vi "Cache.Status.Fglb.vi"(5 "SystemIdx":i32, 7 "Action (get)":T4=enum."get", 8 "error in (no error)":errorcluster, 9 "CheckStatusData":T2, 10 "NewData":T1 {"Values" format="%.3f"}, 11 "Changeover":string) -> (0 "error out":errorcluster, 2 "Data":T3 {"NewData"."Values" format="%.3f"})   [LabVIEW 2016]
uses:
  Cache.Status.Fglb.Action.ctl
  Cache.Status.Fglb.Data.ctl
  Drivers/PLC/LowLevel/PLC.DataBlock.PCcheckstatus.ctl
  Drivers/PLC/LowLevel/PLC.DataBlock.PLCvalues.ctl
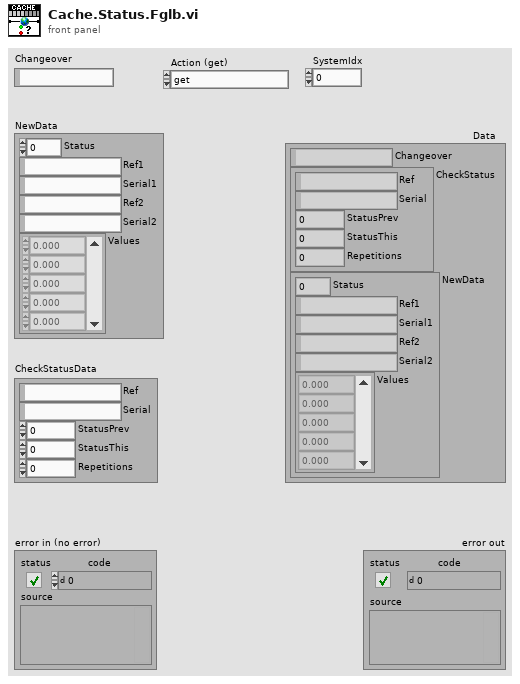
[diagram p1: front panel]
types:
  T1 = typedef "PLC.DataBlock.PLCvalues.ctl" = cluster{"Status":u8, "Ref1":string, "Serial1":string, "Ref2":string, "Serial2":string, "Values":sgl[]}
  T2 = typedef "PLC.DataBlock.PCcheckstatus.ctl" = cluster{"Ref":string, "Serial":string, "StatusPrev":i8, "StatusThis":i8, "Repetitions":u8}
  T3 = typedef "Cache.Status.Fglb.Data.ctl" = cluster{"Changeover":string, "CheckStatus":T2, "NewData":T1}
  T4 = typedef "Cache.Status.Fglb.Action.ctl" = enum16{"init", "Changeover", "CheckStatus", "NewData", "get"}
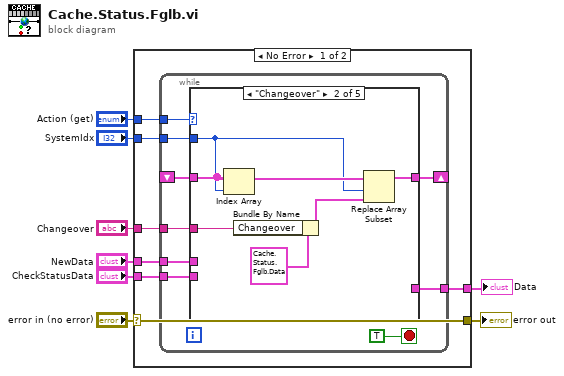
[diagram p0: block diagram]
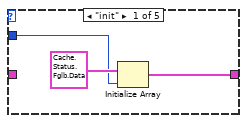
[diagram p2: hidden frame]
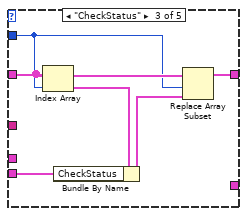
[diagram p3: hidden frame]
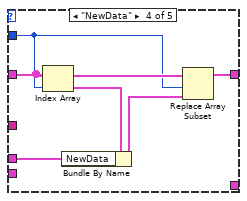
[diagram p4: hidden frame]
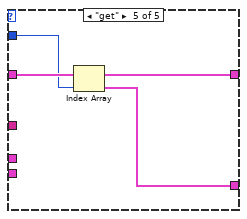
[diagram p5: hidden frame]
diagram:
  n1 = case shown="No Error" "error in (no error)" {
    selector: "error in (no error)" -> [w14 w49]
    tunnel: [w14 w49] -> w7
    tunnel: "Action (get)" -> [w13 _]
    tunnel: "NewData" -> [w15 _]
    tunnel: "SystemIdx" -> [w12 _]
    tunnel: "CheckStatusData" -> [w11 _]
    tunnel: [w10 _] -> w4
    tunnel: "Changeover" -> [w9 _]
    frame No Error {
      n2 = while {
        tunnel: w15 -> [w21]
        tunnel: w13 -> [w24]
        shift-right: [w23] -> _
        shift-left: _ -> [w22]
        tunnel: w12 -> [w19]
        tunnel: w11 -> [w18]
        tunnel: [w17] -> w10
        tunnel: w9 -> [w16]
        stop <- TRUE stop-if-true
        n3 = case shown="\"Changeover\"" w24 {
          tunnel: [w25 w33 w39 w45 w48] -> w23
          tunnel: w22 -> [_ w32 w38 w44 w48]
          tunnel: w21 -> [_ _ _ w40 _]
          tunnel: w19 -> [w26 w31 w36 w42 w46]
          tunnel: w18 -> [_ _ w34 _ _]
          tunnel: [_ _ _ _ w47] -> w17
          tunnel: w16 -> [_ w29 _ _ _]
          frame "init" {
            n4 = Initialize Array(T3 {"Changeover"="", "CheckStatus"={"Ref"="", "Serial"="", "StatusPrev"=0, "StatusThis"=0, "Repetitions"=0}, "NewData"={"Status"=0, "Ref1"="", "Serial1"="", "Ref2"="", "Serial2"="", "Values"=[]}} ("Data"), w26) -> (w25:T3[])
          }
          frame "Changeover" {
            n5 = Index Array(array=w32, index=w31) -> ()  [unwired: 1 out]
            n6 = Bundle By Name(cluster=T3 {"Changeover"="", "CheckStatus"={"Ref"="", "Serial"="", "StatusPrev"=0, "StatusThis"=0, "Repetitions"=0}, "NewData"={"Status"=0, "Ref1"="", "Serial1"="", "Ref2"="", "Serial2"="", "Values"=[]}} ("element"), "Changeover"=w29) -> (w30:T3)
            n7 = Replace Array Subset(array=w32, new element=w30, index=w31) -> (w33:T3[])
          }
          frame "CheckStatus" {
            n8 = Index Array(array=w38, index=w36) -> (element=w35:T3)
            n9 = Bundle By Name(cluster=w35, "CheckStatus"=w34) -> (w37:T3)
            n10 = Replace Array Subset(array=w38, new element=w37, index=w36) -> (w39:T3[])
          }
          frame "NewData" {
            n11 = Index Array(array=w44, index=w42) -> (element=w41:T3)
            n12 = Bundle By Name(cluster=w41, "NewData"=w40) -> (w43:T3)
            n13 = Replace Array Subset(array=w44, new element=w43, index=w42) -> (w45:T3[])
          }
          frame "get" {
            n14 = Index Array(array=w48, index=w46) -> (element=w47:T3)
          }
        }
      }
    }
    frame Error {
    }
  }
  "error out" <- w7
  "Data" <- w4
